vi "LogitechF310_JoyStick_map.vi"(0 "JoystickDevRef":T3) -> (1 "AxesCluster":T2, 2 "ButtonsCluster":T1)   [LabVIEW 2014]
uses:
  <vilib>/Rock Robotics/WPI/Joystick/WPI_JoystickDevRef.ctl
  <vilib>/Rock Robotics/WPI/Joystick/WPI_JoystickDeviceEnum.ctl
  <vilib>/Rock Robotics/Network Tables/SD Write Numeric Array.vi
  <vilib>/Rock Robotics/Network Tables/SD Write Boolean Array.vi
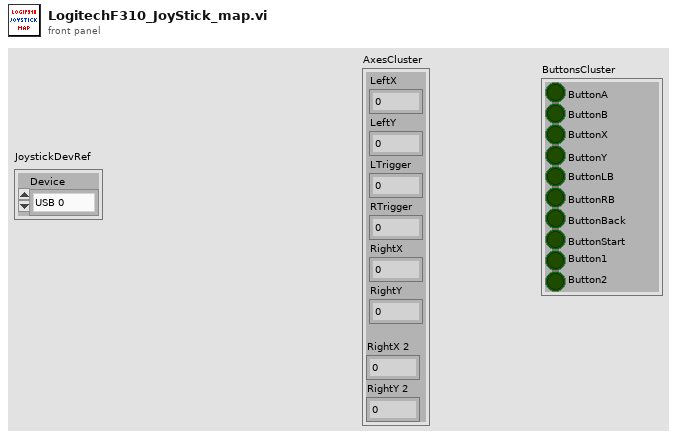
[diagram p1: front panel]
types:
  T1 = cluster{"ButtonA":bool, "ButtonB":bool, "ButtonX":bool, "ButtonY":bool, "ButtonLB":bool, "ButtonRB":bool, "ButtonBack":bool, "ButtonStart":bool, "Button1":bool, "Button2":bool}
  T2 = cluster{"LeftX":dbl, "LeftY":dbl, "LTrigger":dbl, "RTrigger":dbl, "RightX":dbl, "RightY":dbl, "RightY 2":dbl, "RightX 2":dbl}
  T3 = typedef "WPI_JoystickDevRef.ctl" = cluster{"Device":T4}
  T4 = typedef "WPI_JoystickDeviceEnum.ctl" = enum16{"USB 0", "USB 1", "USB 2", "USB 3", "USB 4", "USB 5"}
  T5 = cluster{"upper limit":dbl, "upper limit":dbl, "upper limit":dbl, "upper limit":dbl, "upper limit":dbl, "upper limit":dbl, "upper limit":dbl, "upper limit":dbl}
  T6 = cluster{bool, bool, bool, bool, bool, bool, bool, bool, bool, bool}
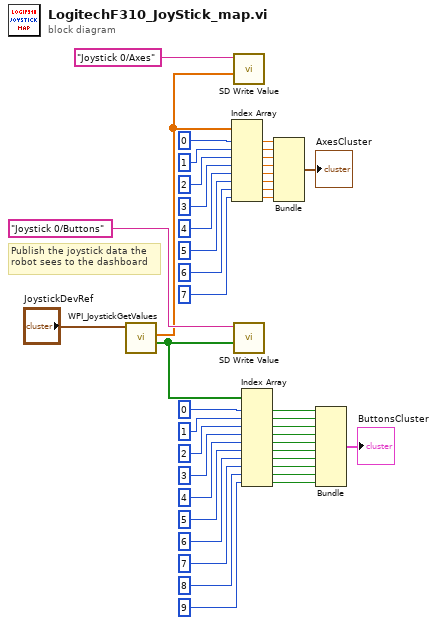
[diagram p0: block diagram]
diagram:
  # "Publish the joystick data the\nrobot sees to the dashboard"
  n1 = call <vilib>:"WPI_JoystickGetValues.vi"("JoystickDevRef"="JoystickDevRef") -> ("Buttons"=w37:bool[], "Axes"=w42:dbl[])  [unwired: 6 in, 3 out]
  n2 = Index Array(array=w42, index #1=0, index #2=1, index #3=2 ("index"), index #4=3 ("index"), index #5=4 ("index"), index #6=5 ("index"), index #7=6, index #8=7) -> (element #1=w24:dbl, element #2=w23:dbl, element #3=w22:dbl, element #4=w21:dbl, element #5=w18:dbl, element #6=w17:dbl, element #7=w2:dbl, element #8=w1:dbl)
  n3 = call-poly <vilib>:"SD Write Value.vi"("Numeric Array"=w42, "Name"="Joystick 0/Axes") -> ()  [unwired: 8 in, 2 out]
  n4 = call-poly <vilib>:"SD Write Value.vi"("Boolean Array"=w37, "Name"="Joystick 0/Buttons") -> ()  [unwired: 8 in, 2 out]
  n5 = Index Array(array=w37, index #1=0, index #2=1, index #3=2 ("index"), index #4=3 ("index"), index #5=4 ("index"), index #6=5 ("index"), index #7=6 ("index"), index #8=7 ("index"), index #9=8 ("index"), index #10=9 ("index")) -> (element #1=w15:bool, element #2=w14:bool, element #3=w13:bool, element #4=w12:bool, element #5=w11:bool, element #6=w10:bool, element #7=w9:bool, element #8=w8:bool, element #9=w7:bool, element #10=w6:bool)
  n6 = Bundle("upper limit"=w24, "upper limit"=w23, "upper limit"=w22, "upper limit"=w21, "upper limit"=w18, "upper limit"=w17, "upper limit"=w2, "upper limit"=w1) -> (→"AxesCluster":T5)  [unwired: 1 in]
  n7 = Bundle(w15, w14, w13, w12, w11, w10, w9, w8, w7, w6) -> (→"ButtonsCluster":T6)  [unwired: 1 in]
